vi "Set Mock as Parent.vi"(8 "error in (no error)":errorcluster, 11 "Mock Class Generator in":refnum<class "Pure Mock Class Generator.lvclass">) -> (0 "error out":errorcluster, 3 "Mock Class Generator out":refnum<class "Pure Mock Class Generator.lvclass">)   [LabVIEW 2020, in "Pure Mock Class Generator.lvclass"]
uses:
  Pure Mock Class Generator.lvclass
  Pure Mock Class Generator.lvclass/Pure Mock Class Generator.ctl
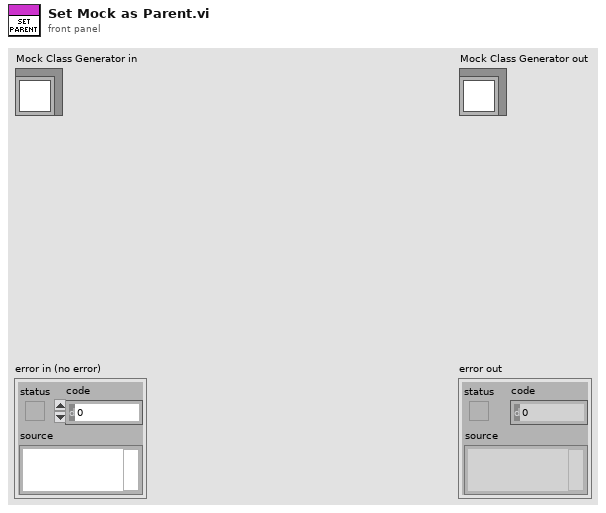
[diagram p1: front panel]
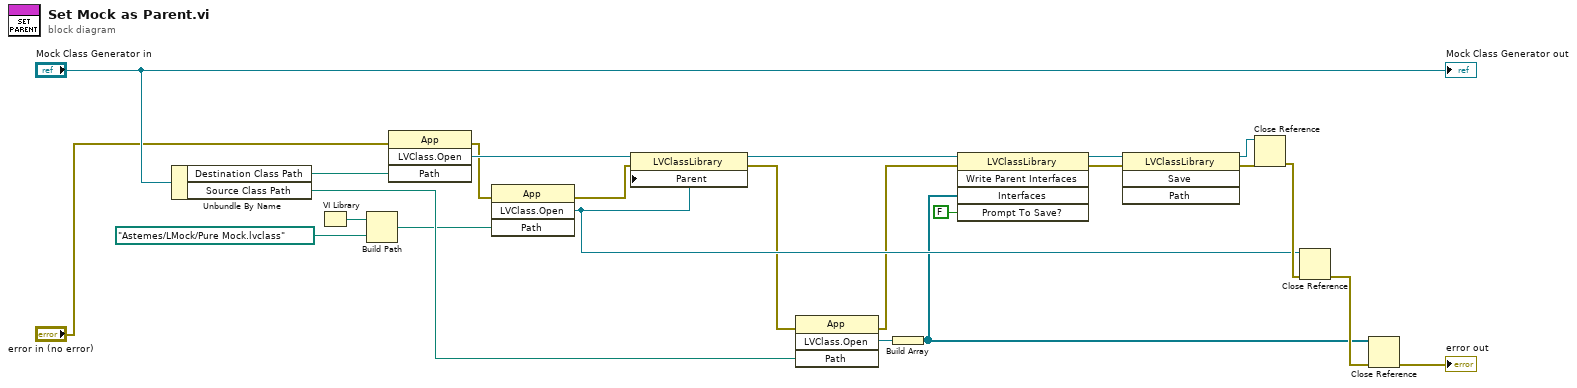
[diagram p0: block diagram]
diagram:
  n1 = Unbundle By Name("Mock Class Generator in") -> ("Destination Class Path"=w22:path, "Source Class Path"=w6:path)
  n2 = VI Library() -> (path=w1:path)
  n3 = Build Path(base path=w1, name or relative path=path "Astemes/LMock/Pure Mock.lvclass" ("class path")) -> (appended path=w2:path)
  n4 = invoke class="App" method="LVClass.Open"(error in="error in (no error)", "Path"=w22) -> (error out=w18:errorcluster, "LVClass.Open"=w21:refnum<vi>)  [unwired: 2 in, 2 out]
  n5 = invoke class="App" method="LVClass.Open"(error in=w18, "Path"=w2) -> (error out=w24:errorcluster, "LVClass.Open"=w19:refnum<vi>)  [unwired: 2 in, 2 out]
  n6 = property class="LVClassLibrary"(reference=w21, error in=w24, "Parent"=w19) -> (reference out=w12:refnum<vi>, error out=w9:errorcluster)
  n7 = invoke class="App" method="LVClass.Open"(error in=w9, "Path"=w6) -> (error out=w8:errorcluster, "LVClass.Open"=w7:refnum<vi>)  [unwired: 2 in, 2 out]
  n8 = Build Array(w7) -> (w4:refnum<vi>[])
  n9 = invoke class="LVClassLibrary" method="Write Parent Interfaces"(reference=w12, error in=w8, "Interfaces"=w4, "Prompt To Save?"=FALSE) -> (reference out=w11:refnum<vi>, error out=w13:errorcluster)  [unwired: 1 in, 3 out]
  n10 = invoke class="LVClassLibrary" method="Save"(reference=w11, error in=w13) -> (reference out=w14:refnum<vi>, error out=w15:errorcluster)  [unwired: 2 in, 2 out]
  n11 = Close Reference(reference=w14, error in (no error)=w15) -> (error out=w20:errorcluster)
  n12 = Close Reference(reference=w19, error in (no error)=w20) -> (error out=w16:errorcluster)
  n13 = Close Reference(reference=w4, error in (no error)=w16) -> (error out=→"error out":errorcluster)
  "Mock Class Generator out" <- "Mock Class Generator in"
